vi "MQTT_PubComp_Read.vi"(8 "error in (no error)":errorcluster, 11 "connection ID":refnum<k5>) -> (0 "error out":errorcluster, 2 "Message ID":u16=10 format="%x", 3 "connection ID out":refnum<k5>)   [LabVIEW 2020, in "MQTT_Functions.lvlib"]
doc: "© 2015 - daq.io, LLC - Peter Adelhardt"
uses:
  MQTT_Functions.lvlib
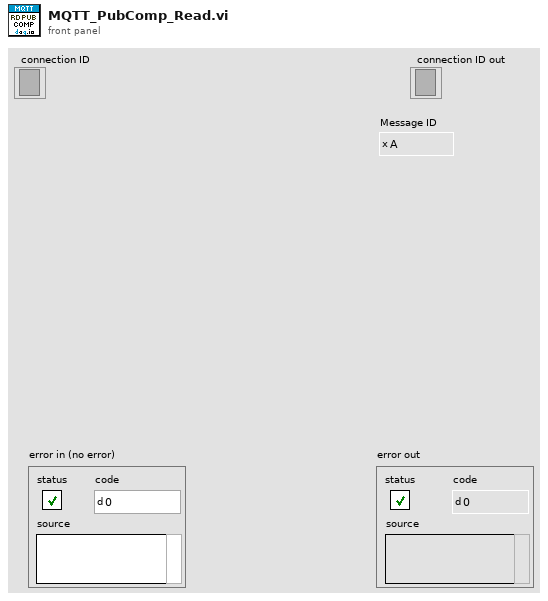
[diagram p1: front panel]
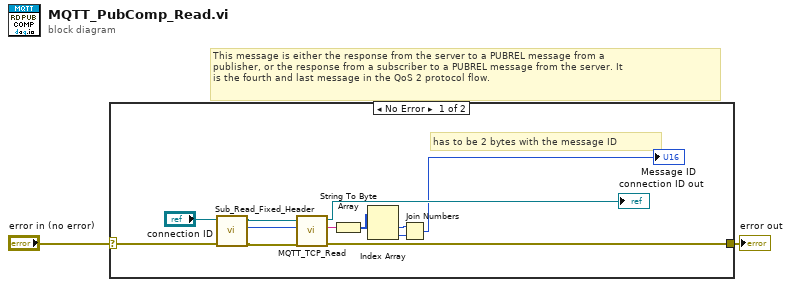
[diagram p0: block diagram]
diagram:
  # "This message is either the response from the server to a PUBREL message from a\npublisher, or the response from a subscriber to a PUBREL message from the server. It\nis the fourth and last message in the QoS 2 protocol flow."
  n1 = case shown="No Error" "error in (no error)" {
    selector: "error in (no error)" -> [w7 w15]
    tunnel: [w6 w15] -> w1
    frame No Error {
      # "has to be 2 bytes with the message ID"
      n2 = call "Sub_Read_Fixed_Header.vi"("error in (no error)"=w7, "connection ID"="connection ID") -> ("error out"=w3:errorcluster, "Remaining Length"=w5:u32, "connection ID out"=w4:refnum<k5>)  [unwired: 3 in, 4 out]
      n3 = call "MQTT_TCP_Read.vi"("error in (no error)"=w3, "bytes to read"=w5, "connection ID"=w4) -> ("error out"=w6:errorcluster, "data out"=w14:string, "connection ID out"=→"connection ID out":refnum<k5>)  [unwired: 6 in]
      n4 = String To Byte Array(string=w14) -> (unsigned byte array=w13:u8[])
      n5 = Index Array(array=w13) -> (element #1=w9:u8, element #2=w10:u8)  [unwired: 2 in]
      n6 = Join Numbers(hi=w9, lo=w10) -> ((hi.lo)=→"Message ID":u16)
    }
    frame Error {
    }
  }
  "error out" <- w1
